vi "量程参数设置对话框.vi"(11 "量程参数":T1={"水温 (℃)"={"量程下限"=0.0, "量程上限"=60.0}, "DO (mg/L)"={"量程下限"=0.0, "量程上限"=25.0}, "DO (%)"={"量程下限"=0.0, "量程上限"=250.0}, "pH"={"量程下限"=0.0, "量程上限"=14.0}, "电导率 (μS/cm)"={"量程下限"=0.0, "量程上限"=100000.0}, "盐度"={"量程下限"=0.0, "量程上限"=50.0}, "浊度 (NTU)"={"量程下限"=0.0, "量程上限"=1000.0}, "叶绿素a (μg/L)"={"量程下限"=0.0, "量程上限"=500.0}, "藻密度 (cells/mL)"={"量程下限"=0.0, "量程上限"=200000.0}, "ORP (mV)"={"量程下限"=-1999.0, "量程上限"=1999.0}}) -> (2 "布尔":bool, 3 "量程参数 2":T1={"水温 (℃)"={"量程下限"=0.0, "量程上限"=60.0}, "DO (mg/L)"={"量程下限"=0.0, "量程上限"=25.0}, "DO (%)"={"量程下限"=0.0, "量程上限"=250.0}, "pH"={"量程下限"=0.0, "量程上限"=14.0}, "电导率 (μS/cm)"={"量程下限"=0.0, "量程上限"=100000.0}, "盐度"={"量程下限"=0.0, "量程上限"=50.0}, "浊度 (NTU)"={"量程下限"=0.0, "量程上限"=1000.0}, "叶绿素a (μg/L)"={"量程下限"=0.0, "量程上限"=500.0}, "藻密度 (cells/mL)"={"量程下限"=0.0, "量程上限"=200000.0}, "ORP (mV)"={"量程下限"=-1999.0, "量程上限"=1999.0}})   [LabVIEW 2016, in "斯坦道多参数.lvlib"]
panel:
  in  "量程参数表":i32(listbox)
  in  "取消":bool
  in  "确认":bool
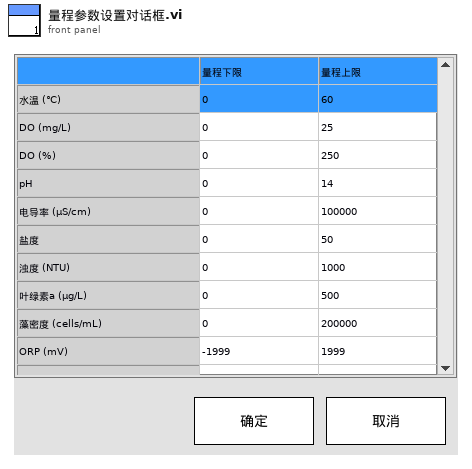
[diagram p1: front panel]
types:
  T1 = cluster{"水温 (℃)":cluster{"量程下限":dbl, "量程上限":dbl}, "DO (mg/L)":cluster{"量程下限":dbl, "量程上限":dbl}, "DO (%)":cluster{"量程下限":dbl, "量程上限":dbl}, "pH":cluster{"量程下限":dbl, "量程上限":dbl}, "电导率 (μS/cm)":cluster{"量程下限":dbl, "量程上限":dbl}, "盐度":cluster{"量程下限":dbl, "量程上限":dbl}, "浊度 (NTU)":cluster{"量程下限":dbl, "量程上限":dbl}, "叶绿素a (μg/L)":cluster{"量程下限":dbl, "量程上限":dbl}, "藻密度 (cells/mL)":cluster{"量程下限":dbl, "量程上限":dbl}, "ORP (mV)":cluster{"量程下限":dbl, "量程上限":dbl}}
  T2 = typedef "LVPoint32TypeDef.ctl" = cluster{"Horizontal":i32, "Vertical":i32}
  T3 = typedef "LVRowAndColumnTypeDef.ctl" = cluster{"Row":i32, "Column":i32}
  T4 = cluster{"[0]":cluster{"[0]":dbl, "[1]":dbl}, "[1]":cluster{"[0]":dbl, "[1]":dbl}, "[2]":cluster{"[0]":dbl, "[1]":dbl}, "[3]":cluster{"[0]":dbl, "[1]":dbl}, "[4]":cluster{"[0]":dbl, "[1]":dbl}, "[5]":cluster{"[0]":dbl, "[1]":dbl}, "[6]":cluster{"[0]":dbl, "[1]":dbl}, "[7]":cluster{"[0]":dbl, "[1]":dbl}, "[8]":cluster{"[0]":dbl, "[1]":dbl}, "[9]":cluster{"[0]":dbl, "[1]":dbl}}
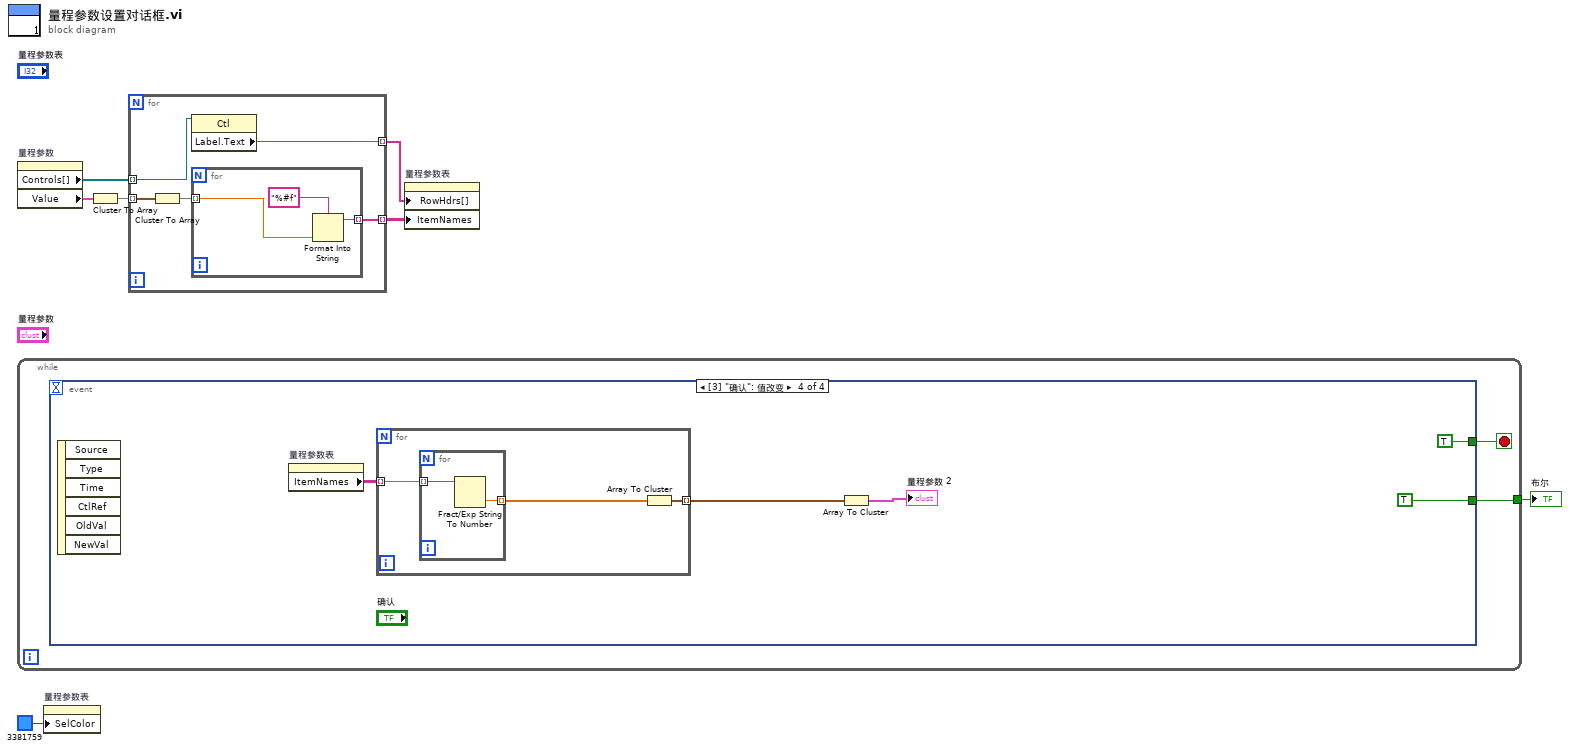
[diagram p0: block diagram]
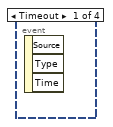
[diagram p2: hidden frame]
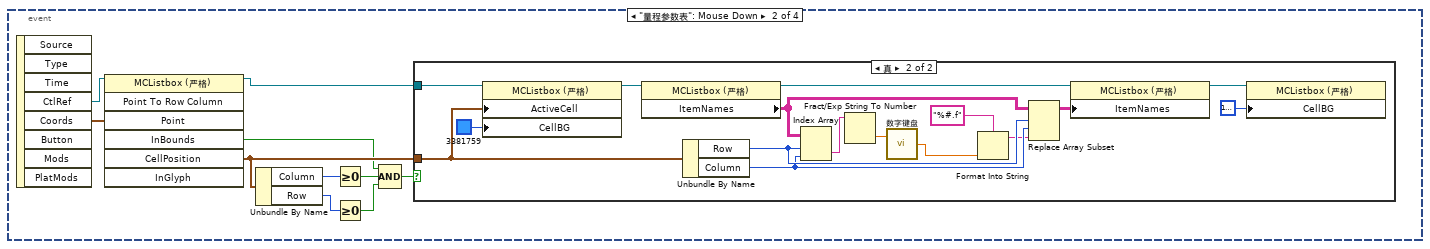
[diagram p3: hidden frame]
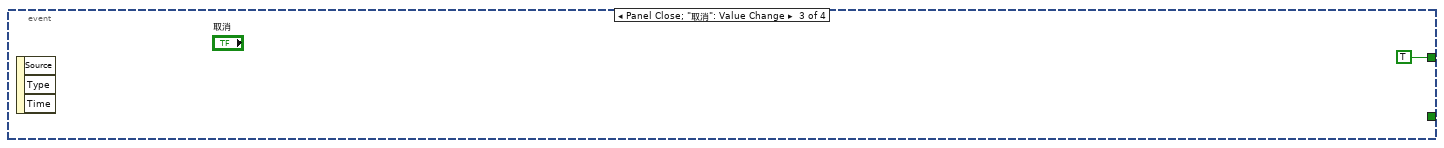
[diagram p5: hidden frame]
diagram:
  n1 = property on="量程参数" class="Clust (严格)"() -> ("Controls[]"=w5:refnum<vi>[], "Value"=w4:T1)  [unwired: 2 in, 2 out]
  n2 = while {
    tunnel: [w8] -> w1
    stop <- w9 stop-if-true
    n3 = event shown="[3] \"确认\": 值改变" {
      selector: _ -> [_ _ _ _]
      dyn-events: _ -> [_ _ _ _]
      timeout: _ -> [_ _ _ _]
      tunnel: [_ _ TRUE TRUE] -> w9
      tunnel: [_ _ _ TRUE] -> w8
      event Timeout {
        n4 = event-data() -> ()  [unwired: 1 in, 3 out]
      }
      event "量程参数表": Mouse Down {
        n5 = event-data() -> ("CtlRef"=w19:refnum<vi>, "Coords"=w18:T2)  [unwired: 1 in, 6 out]
        n6 = invoke class="MCListbox (严格)" method="Point To Row Column"(reference=w19, "Point"=w18) -> (reference out=w17:refnum<vi>, "InBounds"=w13:bool, "CellPosition"=w16:T3)  [unwired: 5 in, 4 out]
        n7 = Unbundle By Name(w16) -> ("Column"=w15:i32, "Row"=w14:i32)
        n8 = Greater Or Equal To 0?(x=w15) -> (x >= 0?=w12:bool)
        n9 = Greater Or Equal To 0?(x=w14) -> (x >= 0?=w11:bool)
        n10 = Compound Arithmetic op=AND ("复合运算")(w13, w12, w11) -> (w10:bool)
        n11 = case shown="真" w10 {
          tunnel: w17 -> [_ w25]
          tunnel: w16 -> [_ w22]
          frame False {
          }
          frame True {
            n12 = property class="MCListbox (严格)"(reference=w25, "ActiveCell"=w22, "CellBG"=u32 3381759 ("活动单元格:单元格背景色")) -> (reference out=w24:refnum<vi>)  [unwired: 1 in, 1 out]
            n13 = property class="MCListbox (严格)"(reference=w24) -> (reference out=w35:refnum<vi>, "ItemNames"=w33:string[][])  [unwired: 1 in, 1 out]
            n14 = Unbundle By Name(w22) -> ("Row"=w32:i32, "Column"=w31:i32)
            n15 = Index Array(array=w33, index (row)=w32, index (col)=w31) -> (element=w30:string)
            n16 = Fract/Exp String To Number(string=w30) -> (number=w29:dbl)  [unwired: 3 in, 1 out]
            n17 = call "数字键盘.vi"("OldNumber"=w29) -> ("NewNumber"=w28:dbl)  [unwired: 1 in]
            n18 = Format Into String(format string="%#.f" ("格式字符串"), w28) -> (resulting string=w26:string)  [unwired: 2 in, 1 out]
            n19 = Replace Array Subset(array=w33, new element=w26, index (row)=w32, index (col)=w31) -> (w34:string[][])
            n20 = property class="MCListbox (严格)"(reference=w35, "ItemNames"=w34) -> (reference out=w23:refnum<vi>)  [unwired: 1 in, 1 out]
            n21 = property class="MCListbox (严格)"(reference=w23, "CellBG"=u32 16777225 ("活动单元格:单元格背景色")) -> ()  [unwired: 1 in, 2 out]
          }
        }
      }
      event Panel Close; "取消": Value Change {
        n22 = event-data() -> ()  [unwired: 1 in, 3 out]
      }
      event "确认": Value Change {
        n23 = event-data() -> ()  [unwired: 1 in, 6 out]
        n24 = property on="量程参数表" class="MCListbox (严格)"() -> ("ItemNames"=w41:string[][])  [unwired: 2 in, 2 out]
        n25 = for {
          tunnel: w41 -> [w44] mode=indexing
          tunnel: [w42] -> w40 mode=indexing
          n26 = for {
            tunnel: w44 -> [w46] mode=indexing
            tunnel: [w45] -> w43 mode=indexing
            n27 = Fract/Exp String To Number(string=w46) -> (number=w45:dbl)  [unwired: 3 in, 1 out]
          }
          n28 = Array To Cluster(array=w43) -> (cluster=w42:cluster{"[0]":dbl, "[1]":dbl})
        }
        n29 = Array To Cluster(array=w40) -> (cluster=→"量程参数 2":T4)
      }
    }
  }
  "布尔" <- w1
  n30 = property on="量程参数表" class="MCListbox (严格)"("SelColor"=u32 3381759 ("活动单元格:单元格背景色")) -> ()  [unwired: 2 in, 2 out]
  n31 = Cluster To Array(cluster=w4) -> (array=w7:cluster{"量程下限":dbl, "量程上限":dbl}[])
  n32 = for {
    tunnel: w7 -> [w51] mode=indexing
    tunnel: [w48] -> w6 mode=indexing
    tunnel: w5 -> [w49] mode=indexing
    tunnel: [w47] -> w3 mode=indexing
    n33 = Cluster To Array(cluster=w51) -> (array=w50:dbl[])
    n34 = property class="Ctl"(reference=w49) -> ("Label.Text"=w47:string)  [unwired: 1 in, 2 out]
    n35 = for {
      tunnel: w50 -> [w54] mode=indexing
      tunnel: [w52] -> w48 mode=indexing
      n36 = Format Into String(format string="%#f" ("格式字符串"), w54) -> (resulting string=w52:string)  [unwired: 2 in, 1 out]
    }
  }
  n37 = property on="量程参数表" class="MCListbox (严格)"("RowHdrs[]"=w3, "ItemNames"=w6) -> ()  [unwired: 2 in, 2 out]
